vi "Create ClusterQueue.vi"(7 "Initial Commands":string[](array[string]), 8 "error in":errorcluster, 11 "Queue Name":string) -> (0 "error out":errorcluster, 3 "Queue Out":refnum<queue>)   [LabVIEW 2010]
doc: "This VI creates a new queue that consists of a cluster of elements. The cluster is a command (string) and data (variant). It also allows initialization of the queue with input commands.\n\nInputs:\nQueue Name - Name of the queue to be created\nInitial Commands - Commands to place in the queue after creation.\nerror in - error input cluster\n\nOutputs:\nQueue Out - create queue reference\nerror out - error output cluster"
uses:
  <userlib>/Common/Queue with Cluster/TYP_Queue Cluster Element.ctl
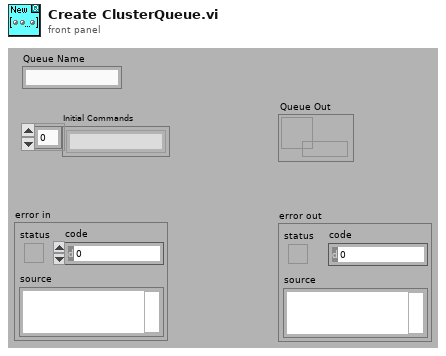
[diagram p1: front panel]
types:
  T1 = typedef "TYP_Queue Cluster Element.ctl" = cluster{"Command":string, "Data":variant}
  T2 = typedef "TYP_Queue with Cluster Reference.ctl" = refnum<queue>
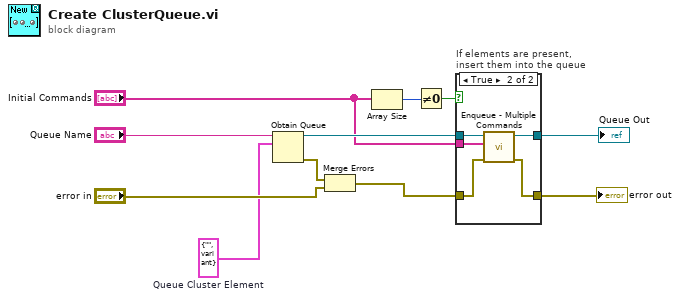
[diagram p0: block diagram]
diagram:
  w7 = T1 {"Command"="", "Data"=variant}  # Queue Cluster Element
  n1 = Obtain Queue(name (unnamed)="Queue Name", element data type=w7) -> (queue out=w5:refnum<queue>, error out=w6:errorcluster)  [unwired: 3 in, 1 out]
  n2 = Merge Errors(w6, "error in") -> (w4:errorcluster)
  n3 = Array Size(array="Initial Commands") -> (size(s)=w2:i32)
  n4 = Not Equal To 0?(x=w2) -> (x != 0?=w1:bool)
  n5 = case "If elements are present,\ninsert them into the queue" shown="True" w1 {
    tunnel: [w12 w18] -> w11
    tunnel: [w13 w17] -> w8
    tunnel: w5 -> [w13 w16]
    tunnel: w4 -> [w12 w15]
    tunnel: "Initial Commands" -> [_ w14]
    frame False {
    }
    frame True {
      n6 = call <userlib>:"Enqueue - Multiple Commands.vi"("error in"=w15, "Array of Commands"=w14, "Queue with Cluster Reference"=w16) -> ("error out"=w18:errorcluster, "Queue (dup)"=w17:T2)  [unwired: 7 in]
    }
  }
  "error out" <- w11
  "Queue Out" <- w8
